vi "Bertta_v09_91.vi"() -> ()   [LabVIEW 2015]
panel:
  out "element":bool
  out "Started:":string
  in  "SHUTDOWN":bool
  in  "MASTER CONTROL":bool
  in  "Tab Control":T1(tab)
  out "Output File":path caption="selected path"
  in  "Browse folder":path=path "" caption="start path"
  in  "Read Seq":bool
  in  "Save Seq":bool
  in  "Configuration file":path=path "C:/Users/shresplab/Desktop/BerttaConfiguration.lvm" caption="Filename"
  in  "OK Button 2":bool
  out "Boolean":bool
  in  "User (initials)":string
  in  "Project name":string
  in  "Description":string
  out "PUMP1":bool
  out "Target amount":dbl
  out "Scale weight":dbl
  out "Amount now":dbl
  out "Flow rate":dbl
  out "Time to target":dbl format="%<%H:%M:%S>t"
  out "Current step":dbl
  out "Target":dbl
  out "Amount now":dbl
  out "Amount now":dbl
  out "Target":dbl
  out "Current step":dbl
  out "Time to target":dbl format="%<%H:%M:%S>t"
  out "Flow rate":dbl
  out "Amount now":dbl
  out "Scale weight":dbl
  out "Target amount":dbl
  out "PUMP2":bool
  out "Sensor OK 6":bool
  out "Sensor OK 5":bool
  out "Sensor OK 4":bool
  out "Sensor OK 3":bool
  in  "OK Button":bool
  in  "Add comment":string
  out "PUMP3":bool
  out "Target amount":dbl
  out "Scale weight":dbl
  out "Amount now":dbl
  out "Flow rate":dbl
  out "Time to target":dbl format="%<%H:%M:%S>t"
  out "Current step":dbl
  out "Target":dbl
  out "Amount now":dbl
  out "Tr":dbl
  out "Tj in":dbl
  out "Tj out":dbl
  out "T set":dbl
  out "Current step":i32
  out "RPM":dbl
  out "Torque 2":dbl
  out "Waveform Chart 5":dynamicdata(graph)
  out "Waveform Chart 6":dynamicdata(graph)
  out "Waveform Chart 7":dynamicdata(graph)
  in  "Tab Control 2":T2(tab)
  out "Waveform Chart 3":dynamicdata(graph)
  out "Waveform Chart 8":dynamicdata(graph)
  out "Waveform Chart 11":dynamicdata(graph)
  out "Waveform Chart 13":dynamicdata(graph)
  out "Waveform Chart 9":dynamicdata(graph)
  out "Table":string[][](table)=[["14.8.2017 18.06.59", "0,000000", "417,670000", "-0,150000", "1,000000", "22,220000", "23,366837", "23,574959", "23,985852", "23,690000", "240,000000", "4,000000", "0,000000", "397,000000", "-397,000000", "1,000000"], ["14.8.2017 18.07.06", "0,000000", "417,640000", "-0,120000", "1,000000", "22,220000", "23,763115", "23,906257", "23,985694", "23,680000", "240,000000", "4,000000", "0,000000", "397,000000", "-397,000000", "1,000000"], ["14.8.2017 18.07.13", "0,000000", "417,640000", "-0,120000", "1,000000", "22,220000", "23,965922", "24,013440", "23,984906", "23,670000", "240,000000", "4,100000", "3,000000", "397,000000", "-397,000000", "1,000000"], ["14.8.2017 18.07.21", "0,000000", "417,640000", "-0,120000", "1,000000", "22,220000", "23,943860", "23,900110", "23,987113", "23,670000", "240,000000", "4,000000", "0,000000", "397,000000", "-397,000000", "1,000000"], ["14.8.2017 18.07.28", "0,000000", "417,640000", "-0,120000", "1,000000", "22,220000", "23,736328", "23,600018", "23,989004", "23,660000", "240,000000", "4,000000", "0,000000", "397,000000", "-397,000000", "1,000000"], ["14.8.2017 18.07.36", "0,000000", "417,640000", "-0,120000", "1,000000", "22,220000", "23,480910", "23,324538", "23,991053", "23,660000", "240,000000", "4,000000", "0,000000", "397,000000", "-397,000000", "1,000000"], ["14.8.2017 18.07.43", "0,000000", "417,640000", "-0,120000", "2,000000", "22,220000", "23,195579", "23,008270", "23,999093", "23,650000", "240,000000", "4,000000", "0,000000", "397,000000", "-397,000000", "1,000000"], ["14.8.2017 18.07.51", "0,000000", "417,650000", "-417,650000", "1,000000", "22,220000", "22,862541", "22,649021", "24,003979", "23,650000", "240,000000", "4,000000", "0,000000", "397,000000", "-397,000000", "2,000000"], ["14.8.2017 18.07.58", "0,000000", "417,640000", "0,010000", "1,000000", "22,220000", "22,541353", "22,354878", "24,005398", "23,650000", "240,000000", "4,000000", "0,000000", "397,000000", "-397,000000", "1,000000"], ["14.8.2017 18.08.06", "0,000000", "417,640000", "0,010000", "1,000000", "22,220000", "22,347931", "22,253738", "24,007605", "23,640000", "240,000000", "4,100000", "0,000000", "397,000000", "-397,000000", "1,000000"], ["14.8.2017 18.08.13", "0,000000", "417,640000", "0,010000", "1,000000", "22,220000", "22,329030", "22,302102", "24,006028", "23,640000", "240,000000", "4,000000", "0,000000", "395,820000", "-395,820000", "1,000000"], ["14.8.2017 18.08.20", "0,000000", "417,640000", "0,010000", "1,000000", "22,220000", "22,466849", "22,511320", "24,002403", "23,630000", "240,000000", "4,000000", "0,000000", "395,830000", "-0,010000", "1,000000"], ["14.8.2017 18.08.28", "0,000000", "417,640000", "0,010000", "1,000000", "22,220000", "22,707062", "22,835101", "24,000984", "23,620000", "240,000000", "4,000000", "0,000000", "395,830000", "-0,010000", "1,000000"], ["14.8.2017 18.08.35", "0,000000", "417,640000", "0,010000", "1,000000", "22,220000", "23,054104", "23,232979", "24,001299", "23,600000", "240,000000", "4,000000", "0,000000", "395,830000", "-0,010000", "1,000000"], ["14.8.2017 18.08.43", "0,000000", "417,640000", "0,010000", "1,000000", "22,220000", "23,412371", "23,522793", "24,002560", "23,590000", "240,000000", "4,000000", "0,000000", "395,820000", "0,000000", "1,000000"], ["14.8.2017 18.08.51", "0,000000", "417,640000", "0,010000", "1,000000", "22,220000", "23,596247", "23,656125", "24,003821", "23,580000", "240,000000", "4,000000", "0,000000", "395,820000", "0,000000", "1,000000"]]
  out "Boolean 2":bool
  in  "Time":dbl format="Time to target (min):                %#_g"
  out "Current temp":dbl format="Current temperature (S1):   %#_6g"
  in  "OK Button 3":bool
  in  "T ext / T ext 2":enum32{"Sensor 1", "Sensor 2"}(radio)
  out "Sensor OK":bool
  in  "T fail":dbl=20.0 format="Failsafe temperature:              %#_g"
  in  "Setpoint":dbl=20.0 format="Temperature target:                %#_6g"
  in  "Manual select":T3(radio)
  in  "PAUSE":bool
  out "Waveform Chart":dynamicdata(graph)
  out "T external 2":dbl format="Current temperature (S2):    %#_g"
  out "Led11 5":bool
  out "RPM":dbl format="%_4f"
  out "Led10 3":bool
  out "Led9 3":bool
  out "Led8 3":bool
  out "Led7 3":bool
  out "Led6 3":bool
  out "Led5 3":bool
  out "Led4 3":bool
  out "Led3 3":bool
  out "Led2 3":bool
  out "Led1 3":bool
  in  "PumpSeq 4":dbl[][](array[numeric])=[[1.0, 1.0, 0.0, 0.0, 0.0, 0.0, 0.0, 0.0, 0.0, 0.0], [2.0, 1.0, 0.0, 0.0, 0.0, 0.0, 0.0, 0.0, 0.0, 0.0], [3.0, 1.0, 0.0, 0.0, 0.0, 0.0, 0.0, 0.0, 0.0, 0.0], [0.0, 0.0, 0.0, 0.0, 0.0, 0.0, 0.0, 0.0, 0.0, 0.0], [0.0, 0.0, 0.0, 0.0, 0.0, 0.0, 0.0, 0.0, 0.0, 0.0], [0.0, 0.0, 0.0, 0.0, 0.0, 0.0, 0.0, 0.0, 0.0, 0.0], [0.0, 0.0, 0.0, 0.0, 0.0, 0.0, 0.0, 0.0, 0.0, 0.0], [0.0, 0.0, 0.0, 0.0, 0.0, 0.0, 0.0, 0.0, 0.0, 0.0], [0.0, 0.0, 0.0, 0.0, 0.0, 0.0, 0.0, 0.0, 0.0, 0.0], [0.0, 0.0, 0.0, 0.0, 0.0, 0.0, 0.0, 0.0, 0.0, 0.0]]
  in  "?":bool
  out "Flow rate (g/min)":dbl
  out "Scale reading":dbl
  out "Step amount now":dbl
  in  "Grams / min":dbl
  out "Waveform Chart 14":dynamicdata(graph)
  in  "?":bool
  out "Total amount now":dbl
  out "Led11 4":bool
  in  "Reset 5":bool
  out "Elapsed / step":i32
  out "Time to target":dbl format="%<%H:%M:%S>t"
  in  "OK Button 4":bool
  out "Led11":bool
  out "RPM":dbl format="%_4f"
  out "Led10":bool
  out "Led9":bool
  out "Led8":bool
  out "Led7":bool
  out "Led6":bool
  out "Led5":bool
  out "Led4":bool
  out "Led3":bool
  out "Led2":bool
  out "Led1":bool
  in  "PumpSeq 2":dbl[][](array[numeric])=[[1.0, 2.0, 0.0, 0.0, 0.0, 0.0, 0.0, 0.0, 0.0, 0.0], [2.0, 2.0, 0.0, 0.0, 0.0, 0.0, 0.0, 0.0, 0.0, 0.0], [3.0, 2.0, 0.0, 0.0, 0.0, 0.0, 0.0, 0.0, 0.0, 0.0], [0.0, 0.0, 0.0, 0.0, 0.0, 0.0, 0.0, 0.0, 0.0, 0.0], [0.0, 0.0, 0.0, 0.0, 0.0, 0.0, 0.0, 0.0, 0.0, 0.0], [0.0, 0.0, 0.0, 0.0, 0.0, 0.0, 0.0, 0.0, 0.0, 0.0], [0.0, 0.0, 0.0, 0.0, 0.0, 0.0, 0.0, 0.0, 0.0, 0.0], [0.0, 0.0, 0.0, 0.0, 0.0, 0.0, 0.0, 0.0, 0.0, 0.0], [0.0, 0.0, 0.0, 0.0, 0.0, 0.0, 0.0, 0.0, 0.0, 0.0], [0.0, 0.0, 0.0, 0.0, 0.0, 0.0, 0.0, 0.0, 0.0, 0.0]]
  in  "?":bool
  out "Flow rate (g/min)":dbl
  out "Scale reading":dbl
  out "Step amount now":dbl
  in  "Grams / min":dbl
  out "Waveform Chart 10":dynamicdata(graph)
  in  "?":bool
  out "Total amount now":dbl
  out "Led11":bool
  in  "Reset 3":bool
  out "Elapsed / step":i32
  out "Time to target":dbl format="%<%H:%M:%S>t"
  in  "OK Button 5":bool
  out "Led11 3":bool
  out "RPM":dbl format="%_4f"
  out "Led10 2":bool
  out "Led9 2":bool
  out "Led8 2":bool
  out "Led7 2":bool
  out "Led6 2":bool
  out "Led5 2":bool
  out "Led4 2":bool
  out "Led3 2":bool
  out "Led2 2":bool
  out "Led1 2":bool
  in  "PumpSeq 3":dbl[][](array[numeric])=[[1.0, 3.0, 0.0, 0.0, 0.0, 0.0, 0.0, 0.0, 0.0, 0.0], [2.0, 3.0, 0.0, 0.0, 0.0, 0.0, 0.0, 0.0, 0.0, 0.0], [3.0, 3.0, 0.0, 0.0, 0.0, 0.0, 0.0, 0.0, 0.0, 0.0], [0.0, 0.0, 0.0, 0.0, 0.0, 0.0, 0.0, 0.0, 0.0, 0.0], [0.0, 0.0, 0.0, 0.0, 0.0, 0.0, 0.0, 0.0, 0.0, 0.0], [0.0, 0.0, 0.0, 0.0, 0.0, 0.0, 0.0, 0.0, 0.0, 0.0], [0.0, 0.0, 0.0, 0.0, 0.0, 0.0, 0.0, 0.0, 0.0, 0.0], [0.0, 0.0, 0.0, 0.0, 0.0, 0.0, 0.0, 0.0, 0.0, 0.0], [0.0, 0.0, 0.0, 0.0, 0.0, 0.0, 0.0, 0.0, 0.0, 0.0], [0.0, 0.0, 0.0, 0.0, 0.0, 0.0, 0.0, 0.0, 0.0, 0.0]]
  in  "?":bool
  out "Flow rate (g/min)":dbl
  out "Scale reading":dbl
  out "Step amount now":dbl
  in  "Grams / min":dbl
  out "Waveform Chart 12":dynamicdata(graph)
  in  "?":bool
  out "Total amount now":dbl
  out "Led11 2":bool
  in  "Reset 4":bool
  out "Elapsed / step":i32
  out "Time to target":dbl format="%<%H:%M:%S>t"
  in  "OK Button 6":bool
  in  "Bypass select 2":enum32{"Remote", "Manual"}(radio)=enum."Manual"
  in  "Port":dbl=13.0
  out "RPM":dbl
  out "Torque":dbl
  in  "Set RPM":dbl(slide) scale=0.0..2000.0
  out "Waveform Chart 4":dynamicdata(graph)
  in  "OK Button 7":bool
  in  "Treshold (T/C)":dbl=0.5
  out "DAQ 9217 (PT100)":errorcluster
  out "Config File":dbl[][](array[numeric])
  # "Temperature sensor:"
  # "Manual control:"
  # "PUMP & SCALE 1"
  # "STEP"
  # "TOTAL"
  # "PUMP & SCALE 2"
  # "STEP"
  # "TOTAL"
  # "PUMP & SCALE 3"
  # "STEP"
  # "TOTAL"
  # "Temperature control parameter"
  # "Secondary temperature sensor"
  # "Grams    /   min"
  # "End of sequence"
  # "Manual control"
  # "Grams    /   min"
  # "End of sequence"
  # "Manual control"
  # "Grams    /   min"
  # "End of sequence"
  # "Manual control"
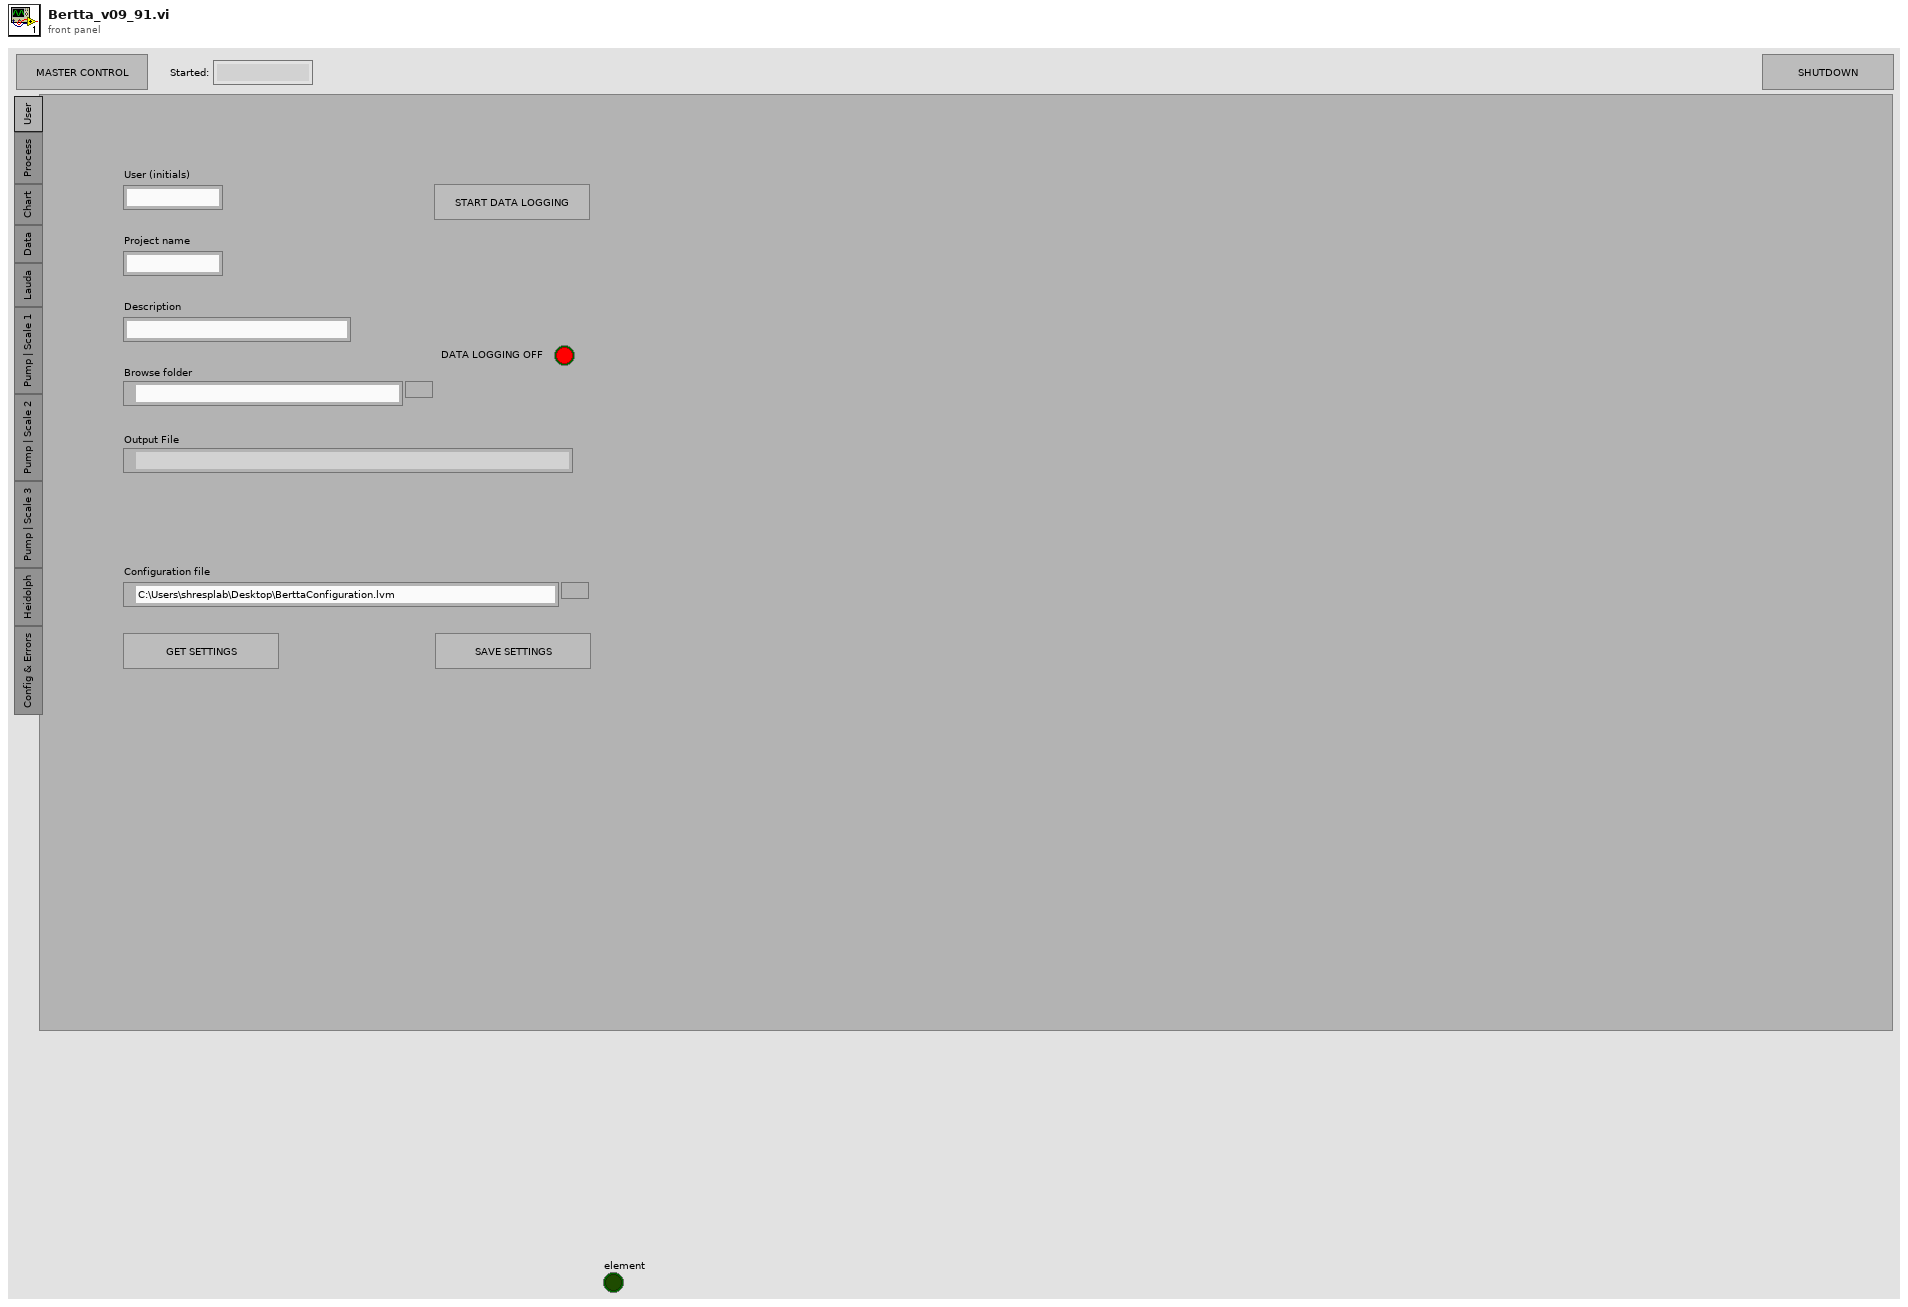
[diagram p1: front panel]
types:
  T1 = enum32{"User", "Process", "Chart", "Data", "Lauda", "Pump | Scale 1", "Pump | Scale 2", "Pump | Scale 3", "Heidolph", "Config & Errors"}
  T2 = enum32{"Temperatures", "Scale / Pump 1", "Scale / Pump 2", "Scale / Pump 3", "RPM / torque"}
  T3 = enum32{"Reactor temperature", "Jacket temperature"}
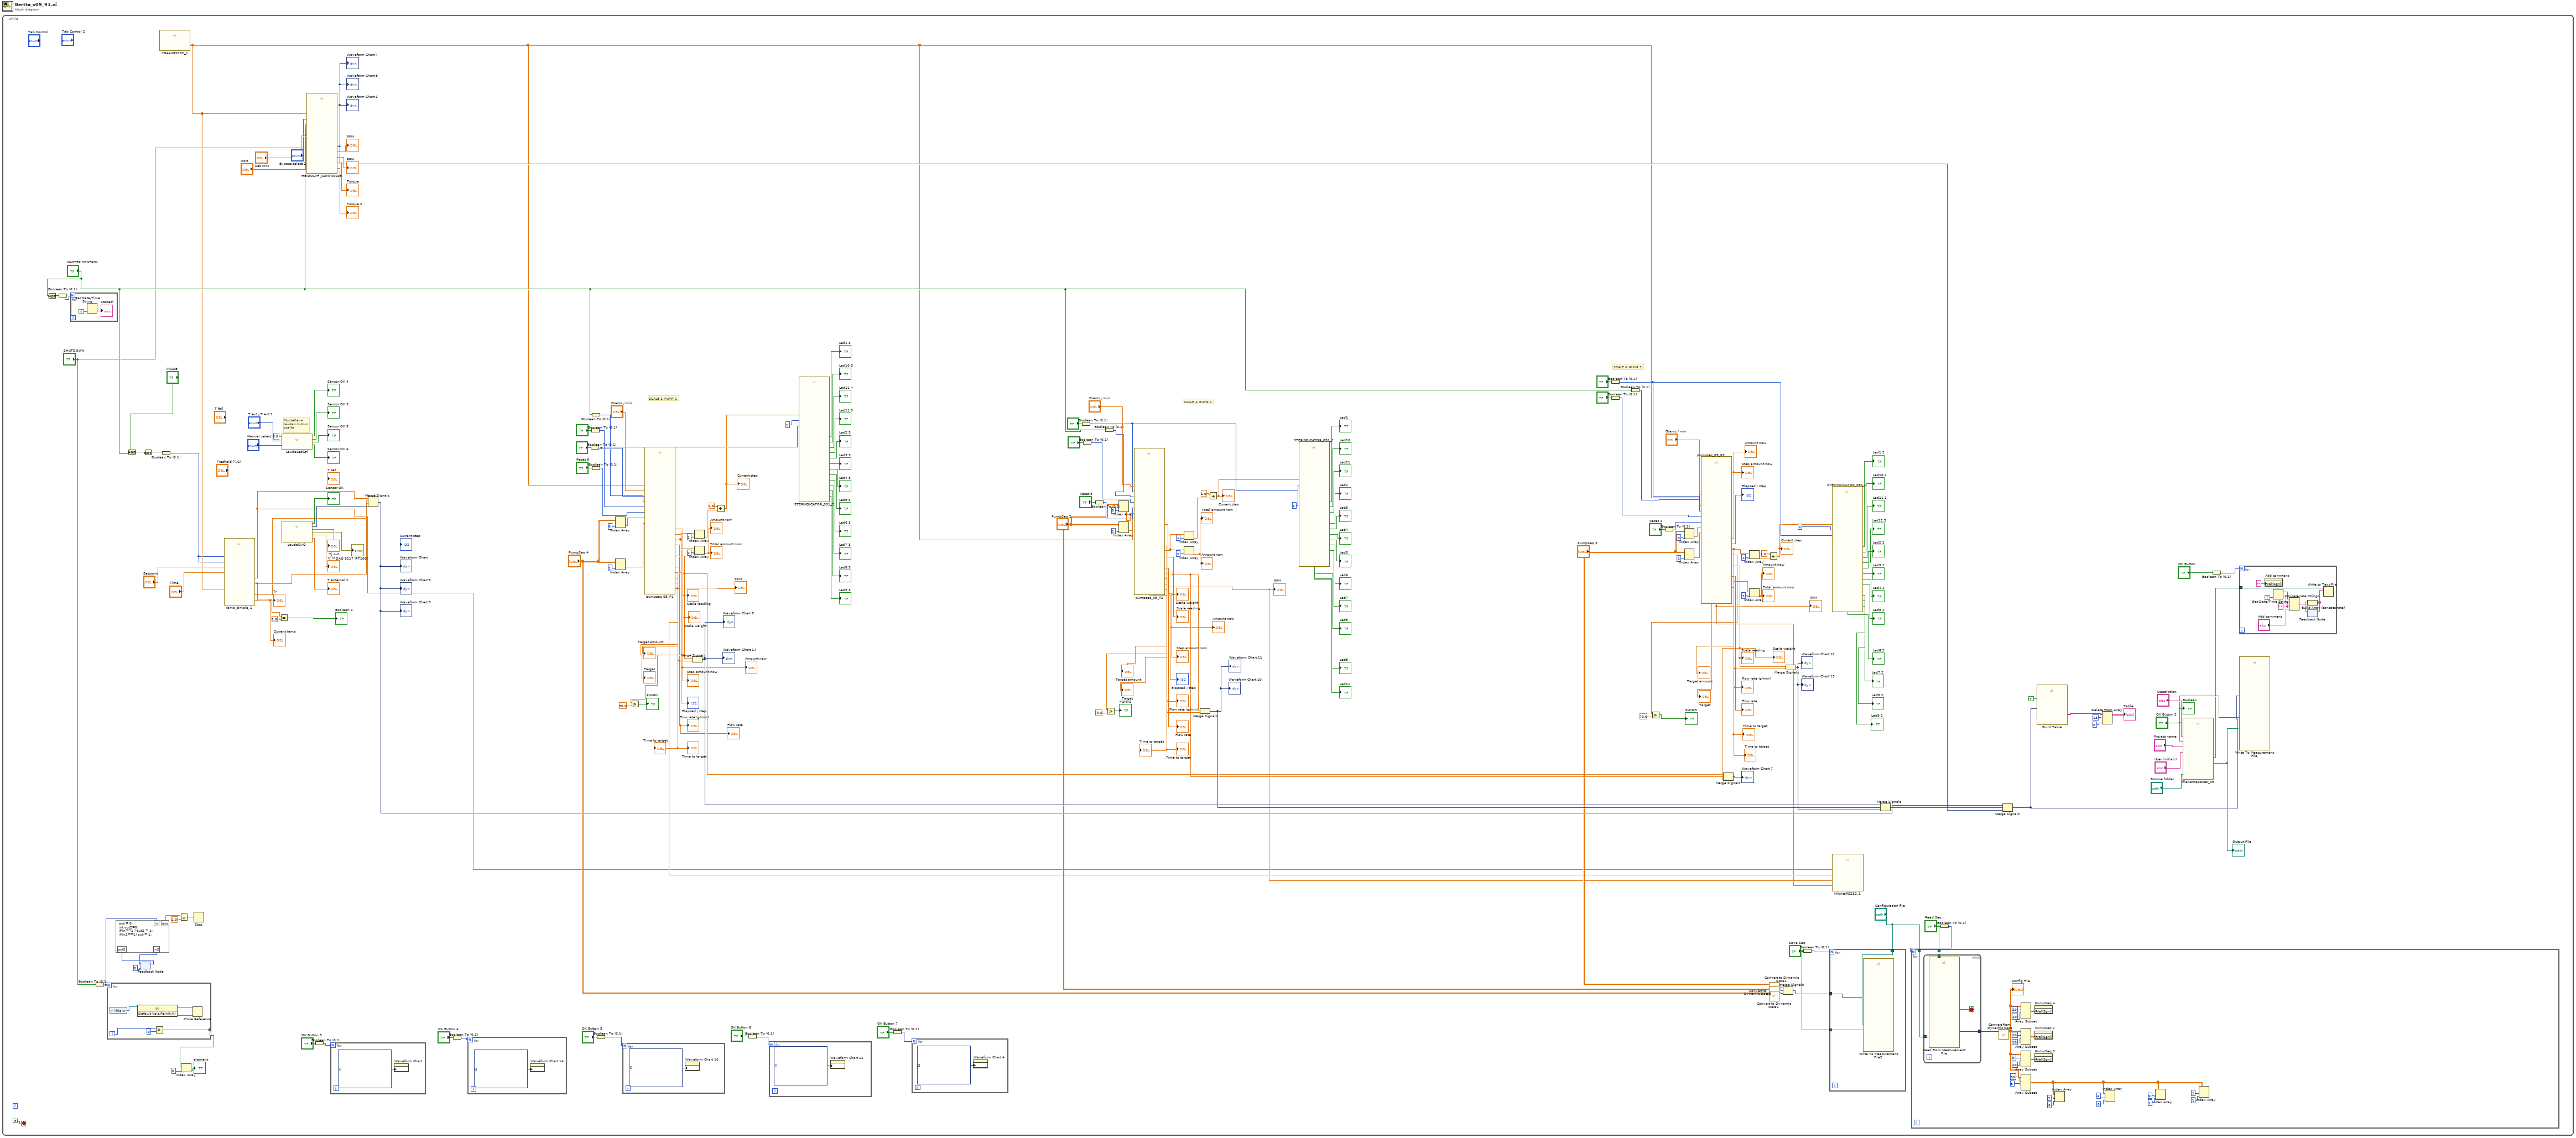
[diagram p0: block diagram]
diagram:
  n1 = while {
    stop <- FALSE stop-if-true
    # "Muutettava\nlaudan kutsun \nosalta"
    # "SCALE & PUMP 1"
    # "SCALE & PUMP 3"
    # "SCALE & PUMP 2"
    n2 = Not(x="MASTER CONTROL") -> (.not. x?=w210:bool)
    n3 = Boolean To (0,1)(Boolean=w210) -> (0, 1=w211:i16)
    n4 = for {
      N: w211 -> [_]
      n5 = Get Date/Time String(want seconds? (F)=TRUE) -> (time string=→"Started:":string)  [unwired: 2 in, 1 out]
    }
    n6 = Boolean To (0,1)(Boolean="SHUTDOWN") -> (0, 1=w193:i16)
    n7 = for {
      N: w193 -> [_]
      tunnel: [w268] -> w209 mode=indexing
      i -> [w270]
      n8 = control-ref of="This VI"() -> (w273:refnum<vi>)
      n9 = invoke class="VI" method="Default Vals.Reinit All"(reference=w273) -> (reference out=w271:refnum<vi>, error out=w272:errorcluster)  [unwired: 2 in, 1 out]
      n10 = Greater?(x=w270, y=0) -> (0:w268:bool)
      n11 = Close Reference(reference=w271, error in (no error)=w272) -> ()  [unwired: 1 out]
    }
    n12 = And(x="PAUSE", y="MASTER CONTROL") -> (x .and. y?=w156:bool)
    n13 = feedback #1(0) -> (w191:i32)
    n14 = formula code="out = 0;\nint out2=0;\nif(in==1 ) out2 = 1;\nif(in2==1) out = 1;"("in"=w193, "in2"=w191) -> ("out"=w195:dbl, "out2"=w192:i32)
    n15 = feedback-in #1(w192) -> ()
    n16 = Not(x=w156) -> (.not. x?=w11:bool)
    n17 = call "MReadRS232_1.vi"() -> ("params"=w8:dbl[])  [unwired: 11 in]
    n18 = Boolean To (0,1)(Boolean=w11) -> (0, 1=w4:i16)
    n19 = Equal?(x=w195, y=1.0) -> (x = y?=w194:bool)
    n20 = Index Array(array=w209, index=0) -> (element=→"element":bool)
    n21 = Stop(stop? (T)=w194) -> ()
    n22 = call "ramp_simple_1.vi"("array"=w8, "time_set"="Time", "T_sp"="Setpoint", "reset"=w4, "pause"=w4) -> ("T control"=w7:dbl, "Tr"=w6:dbl, "Tin"=w5:dbl, "reset_out"=w2:dbl)  [unwired: 3 in]
    "Tr" <- w6
    "Current temp" <- w6
    n23 = Equal?(x=w2, y=1.0) -> (x = y?=→"Boolean 2":bool)
    n24 = call "LaudaLedCtrl.vi"("Manual select"="Manual select", "T ext / T ext in"="T ext / T ext 2", "Lauda port"=9.0) -> ("Sensor OK 5"=→"Sensor OK 5":bool, "Sensor OK 3"=→"Sensor OK 3":bool, "Sensor OK 4"=→"Sensor OK 4":bool, "Sensor OK 6"=→"Sensor OK 6":bool)  [unwired: 5 in]
    n25 = call "LaudaDAQ.vi"() -> ("error out"=→"DAQ 9217 (PT100)":errorcluster, 1:"Tj out"=→"Tj out":dbl, "data"=w79:dynamicdata, "Sensor OK"=→"Sensor OK":bool, 4:"Tj out"=→"Tj in":dbl, "T external 2"=→"T external 2":dbl)  [unwired: 6 in]
    n26 = call "HEIDOLPH_CONTROL09.vi"("master"="MASTER CONTROL", "Array"=w8, "shutdown"="SHUTDOWN", "Bypass select"="Bypass select 2", "Set RPM"="Set RPM", "Device port"="Port") -> ("Dynamic Data"=w80:dynamicdata, "RPM"=→"RPM":dbl, "RPM 2"=→"RPM":dbl, "Torque"=→"Torque":dbl, "Torque 2"=→"Torque 2":dbl)  [unwired: 1 in]
    "Waveform Chart 4" <- w80
    "Waveform Chart 6" <- w80
    "Waveform Chart 9" <- w80
    n27 = Boolean To (0,1)(Boolean="OK Button 3") -> (0, 1=w22:i16)
    n28 = for {
      N: w22 -> [_]
      n29 = property on="Waveform Chart" class="WFChart (strict)"("History Data"=dynamicdata[] []) -> ()  [unwired: 2 in, 2 out]
    }
    n30 = Merge Signals(w7, w6, w5, w79) -> (w81:dynamicdata)
    "Waveform Chart 3" <- w81
    "Waveform Chart" <- w81
    "Waveform Chart 5" <- w81
    n31 = Boolean To (0,1)(Boolean="OK Button 4") -> (0, 1=w20:i16)
    n32 = for {
      N: w20 -> [_]
      n33 = property on="Waveform Chart 14" class="WFChart (strict)"("History Data"=dynamicdata[] []) -> ()  [unwired: 2 in, 2 out]
    }
    n34 = Boolean To (0,1)(Boolean="?") -> (0, 1=w90:i16)
    n35 = Boolean To (0,1)(Boolean="?") -> (0, 1=w94:i16)
    n36 = Boolean To (0,1)(Boolean="MASTER CONTROL") -> (0, 1=w86:i16)
    n37 = Boolean To (0,1)(Boolean="Reset 5") -> (0, 1=w93:i16)
    n38 = Boolean To (0,1)(Boolean="OK Button 5") -> (0, 1=w18:i16)
    n39 = Index Array(array="PumpSeq 4", index (col)=0) -> (element=w98:dbl[])  [unwired: 1 in]
    n40 = Index Array(array="PumpSeq 4", index (col)=1) -> (element=w119:dbl[])  [unwired: 1 in]
    n41 = for {
      N: w18 -> [_]
      n42 = property on="Waveform Chart 10" class="WFChart (strict)"("History Data"=dynamicdata[] []) -> ()  [unwired: 2 in, 2 out]
    }
    n43 = call "pumpsec_09_P1.vi"("reset"=w93, "master"=w86, "manual"=w90, "pause"=w94, "Array"=w8, "Target"=w98, "fr_manual"="Grams / min", "Time"=w119) -> ("pumpCtrl"=w63:dbl, "totaltarget"=→"Target":dbl, "target_step"=→"Target amount":dbl, "REGLO D"=w29:dbl, "time_to_target"=→"Time to target" →"Time to target":dbl, "step_fr"=w40:dbl, "amount_step"=→"Amount now" →"Step amount now":dbl, "Scale"=w75:dbl, "elapsed_step"=→"Elapsed / step":dbl, "params"=w116:dbl[])  [unwired: 8 in, 2 out]
    "Flow rate" <- w40
    "Scale weight" <- w75
    "Scale reading" <- w75
    "Flow rate (g/min)" <- w40
    "RPM" <- w29
    n44 = Greater?(x=w63, y=70.0) -> (0:→"PUMP1":bool)
    n45 = Merge Signals(w75, w40) -> (w84:dynamicdata)
    "Waveform Chart 8" <- w84
    "Waveform Chart 14" <- w84
    n46 = Index Array(array=w116, index=1) -> (element=w113:dbl)
    n47 = Index Array(array=w116, index=2) -> (element=→"Amount now" →"Total amount now":dbl)
    n48 = Add(x=1.0, y=w113) -> (x+y=w41:dbl)
    "Current step" <- w41
    n49 = Boolean To (0,1)(Boolean="OK Button 6") -> (0, 1=w16:i16)
    n50 = for {
      N: w16 -> [_]
      n51 = property on="Waveform Chart 12" class="WFChart (strict)"("History Data"=dynamicdata[] []) -> ()  [unwired: 2 in, 2 out]
    }
    n52 = call "STEPINDICATOR_091_2.vi"("current step"=w41, "enable"=i16 1, "manual"=w90) -> ("Led 8"=→"Led8 3":bool, "Led 10"=→"Led10 3":bool, "Led 11"=→"Led11 4":bool, "Led 7"=→"Led7 3":bool, "Led 1"=→"Led1 3":bool, "Led 6"=→"Led6 3":bool, "Led 2"=→"Led2 3":bool, "Led 12"=→"Led11 5":bool, "Led 5"=→"Led5 3":bool, "Led 4"=→"Led4 3":bool, "Led 3"=→"Led3 3":bool, "Led 9"=→"Led9 3":bool)  [unwired: 1 in]
    n53 = Boolean To (0,1)(Boolean="OK Button 7") -> (0, 1=w14:i16)
    n54 = for {
      N: w14 -> [_]
      n55 = property on="Waveform Chart 4" class="WFChart (strict)"("History Data"=dynamicdata[] []) -> ()  [unwired: 2 in, 2 out]
    }
    n56 = Boolean To (0,1)(Boolean="?") -> (0, 1=w153:i16)
    n57 = Boolean To (0,1)(Boolean="?") -> (0, 1=w182:i16)
    n58 = Boolean To (0,1)(Boolean="Reset 3") -> (0, 1=w180:i16)
    n59 = Boolean To (0,1)(Boolean="MASTER CONTROL") -> (0, 1=w174:i16)
    n60 = Index Array(array="PumpSeq 2", index (col)=0 ("disabled index (col)")) -> (element=w185:dbl[])  [unwired: 1 in]
    n61 = Index Array(array="PumpSeq 2", index (col)=1 ("disabled index (col)")) -> (element=w184:dbl[])  [unwired: 1 in]
    n62 = call "pumpsec_09_P2.vi"("reset"=w180, "master"=w174, "manual"=w153, "pause"=w182, "Array"=w8, "Target"=w185, "fr_manual"="Grams / min", "Time"=w184) -> ("pumpCtrl"=w59:dbl, "totaltarget"=→"Target":dbl, "target_step"=→"Target amount":dbl, "REGLO D"=w28:dbl, "time_to_target"=→"Time to target" →"Time to target":dbl, "step_fr"=w78:dbl, "amount_step"=→"Amount now" →"Step amount now":dbl, "Scale"=w74:dbl, "elapsed_step"=→"Elapsed / step":dbl, "params"=w175:dbl[])  [unwired: 8 in, 2 out]
    "Scale weight" <- w74
    "Flow rate" <- w78
    "Scale reading" <- w74
    "Flow rate (g/min)" <- w78
    "RPM" <- w28
    n63 = Greater?(x=w59, y=70.0) -> (0:→"PUMP2":bool)
    n64 = Index Array(array=w175, index=1) -> (element=w178:dbl)
    n65 = Index Array(array=w175, index=2) -> (element=→"Amount now" →"Total amount now":dbl)
    n66 = Merge Signals(w74, w78) -> (w87:dynamicdata)
    "Waveform Chart 11" <- w87
    "Waveform Chart 10" <- w87
    n67 = Add(x=1.0, y=w178) -> (x+y=w172:dbl)
    "Current step" <- w172
    n68 = call "STEPINDICATOR_091_2.vi"("current step"=w172, "enable"=i16 1, "manual"=w153) -> ("Led 8"=→"Led8":bool, "Led 10"=→"Led10":bool, "Led 11"=→"Led11":bool, "Led 7"=→"Led7":bool, "Led 1"=→"Led1":bool, "Led 6"=→"Led6":bool, "Led 2"=→"Led2":bool, "Led 12"=→"Led11":bool, "Led 5"=→"Led5":bool, "Led 4"=→"Led4":bool, "Led 3"=→"Led3":bool, "Led 9"=→"Led9":bool)  [unwired: 1 in]
    n69 = Boolean To (0,1)(Boolean="?") -> (0, 1=w147:i16)
    n70 = Boolean To (0,1)(Boolean="?") -> (0, 1=w146:i16)
    n71 = Boolean To (0,1)(Boolean="MASTER CONTROL") -> (0, 1=w148:i16)
    n72 = Boolean To (0,1)(Boolean="Reset 4") -> (0, 1=w128:i16)
    n73 = Index Array(array="PumpSeq 3", index (col)=0 ("disabled index (col)")) -> (element=w131:dbl[])  [unwired: 1 in]
    n74 = Index Array(array="PumpSeq 3", index (col)=1 ("disabled index (col)")) -> (element=w130:dbl[])  [unwired: 1 in]
    n75 = call "pumpsec_09_P3.vi"("reset"=w128, "master"=w148, "manual"=w147, "pause"=w146, "Array"=w8, "Target"=w131, "fr_manual"="Grams / min", "Time"=w130) -> ("pumpCtrl"=w56:dbl, "totaltarget"=→"Target":dbl, "target_step"=→"Target amount":dbl, "REGLO D"=w27:dbl, "time_to_target"=→"Time to target" →"Time to target":dbl, "step_fr"=w77:dbl, "amount_step"=→"Amount now" →"Step amount now":dbl, "Scale"=w73:dbl, "elapsed_step"=→"Elapsed / step":dbl, "params"=w121:dbl[])  [unwired: 8 in, 2 out]
    "Scale weight" <- w73
    "Flow rate" <- w77
    "Scale reading" <- w73
    "Flow rate (g/min)" <- w77
    "RPM" <- w27
    n76 = Greater?(x=w56, y=70.0) -> (0:→"PUMP3":bool)
    n77 = Merge Signals(w75, w74, w73) -> (→"Waveform Chart 7":dynamicdata)
    n78 = Index Array(array=w121, index=1) -> (element=w122:dbl)
    n79 = Index Array(array=w121, index=2) -> (element=→"Amount now" →"Total amount now":dbl)
    n80 = Add(x=1.0, y=w122) -> (x+y=w120:dbl)
    "Current step" <- w120
    n81 = call "Convert to Dynamic Data4"("2D Array"="PumpSeq 3") -> ("Dynamic Data Type"=w32:dynamicdata)  [unwired: 3 in]
    n82 = call "Convert to Dynamic Data3"("2D Array"="PumpSeq 2") -> ("Dynamic Data Type"=w34:dynamicdata)  [unwired: 3 in]
    n83 = call "Convert to Dynamic Data2"("2D Array"="PumpSeq 4") -> ("Dynamic Data Type"=w37:dynamicdata)  [unwired: 3 in]
    n84 = Merge Signals(w32, w34, w37) -> (w36:dynamicdata)
    n85 = Merge Signals(w73, w77) -> (w83:dynamicdata)
    "Waveform Chart 13" <- w83
    "Waveform Chart 12" <- w83
    n86 = Boolean To (0,1)(Boolean="Save Seq") -> (0, 1=w31:i16)
    n87 = for {
      N: w31 -> [_]
      tunnel: w36 -> [w266]
      tunnel: "Configuration file" -> [w267]
      tunnel: "Save Seq" -> [w265]
      n88 = call "Write To Measurement File2"("Signals"=w266, "Reset"=w265, "Filename"=w267) -> ()  [unwired: 14 in, 3 out]
    }
    n89 = call "STEPINDICATOR_091_4.vi"("current step"=w120, "enable"=i16 1, "manual"=w147) -> ("Led 8"=→"Led8 2":bool, "Led 10"=→"Led10 2":bool, "Led 11"=→"Led11 2":bool, "Led 7"=→"Led7 2":bool, "Led 1"=→"Led1 2":bool, "Led 6"=→"Led6 2":bool, "Led 2"=→"Led2 2":bool, "Led 12"=→"Led11 3":bool, "Led 5"=→"Led5 2":bool, "Led 4"=→"Led4 2":bool, "Led 3"=→"Led3 2":bool, "Led 9"=→"Led9 2":bool)  [unwired: 1 in]
    n90 = call "MWriteRS232_1.vi"("P3"=w27, "P2"=w28, "P1"=w29, "LAUDA"=w7) -> ()  [unwired: 8 in]
    n91 = Merge Signals(w84, w87, w83) -> (w82:dynamicdata)
    n92 = Boolean To (0,1)(Boolean="Read Seq") -> (0, 1=w30:i16)
    n93 = for {
      N: w30 -> [_]
      tunnel: "Configuration file" -> [w238]
      tunnel: "Read Seq" -> [w237]
      n94 = while {
        tunnel: [w264] -> w260
        tunnel: w238 -> [w263]
        tunnel: w237 -> [w261]
        stop <- w262 stop-if-true
        n95 = call "Read From Measurement File"("Filename"=w263, "Reset"=w261) -> ("Signals"=w264:dynamicdata, "EOF?"=w262:bool)  [unwired: 4 in, 4 out]
      }
      n96 = call "Convert from Dynamic Data"("Dynamic Data Type"=w260) -> ("Array"=w250:dbl[][])  [unwired: 3 in]
      "Config File" <- w250
      n97 = Array Subset(array=w250, index (row)=20 ("index"), length (row)=10 ("length")) -> (w257:dbl[][])  [unwired: 2 in]
      n98 = Array Subset(array=w250, index (row)=10 ("index"), length (row)=10 ("length")) -> (w252:dbl[][])  [unwired: 2 in]
      n99 = Array Subset(array=w250, index (row)=0 ("index"), length (row)=10 ("length")) -> (w251:dbl[][])  [unwired: 2 in]
      n100 = Array Subset(array=w250, index (row)=30 ("index"), length (row)=8 ("length")) -> (w239:dbl[][])  [unwired: 2 in]
      n101 = property on="PumpSeq 4" class="Arr (strict)"("Val(Sgnl)"=w257) -> ()  [unwired: 2 in, 2 out]
      n102 = property on="PumpSeq 2" class="Arr (strict)"("Val(Sgnl)"=w252) -> ()  [unwired: 2 in, 2 out]
      n103 = property on="PumpSeq 3" class="Arr (strict)"("Val(Sgnl)"=w251) -> ()  [unwired: 2 in, 2 out]
      n104 = Index Array(array=w239, index (row)=2, index (col)=0 ("disabled index (col)")) -> ()  [unwired: 1 out]
      n105 = Index Array(array=w239, index (row)=4, index (col)=0 ("disabled index (col)")) -> ()  [unwired: 1 out]
      n106 = Index Array(array=w239, index (row)=0, index (col)=1 ("disabled index (col)")) -> ()  [unwired: 1 out]
      n107 = Index Array(array=w239, index (row)=1, index (col)=1 ("disabled index (col)")) -> ()  [unwired: 1 out]
    }
    n108 = Merge Signals(w81, w82, w80) -> (w204:dynamicdata)
    n109 = call "Build Table"("Include time data"=TRUE, "Signals"=w204) -> ("Table"=w203:string[][])  [unwired: 3 in, 6 out]
    n110 = Delete From Array(array=w203, length=13, index (col)=0 ("index (row)")) -> (array with subset deleted=→"Table":string[][])  [unwired: 1 in, 1 out]
    n111 = call "filenameparser_09.vi"("Description"="Description", "start path"="Browse folder", "Project name"="Project name", "User (initials)"="User (initials)", "OK Button in"="OK Button 2") -> ("appended path 2"=w12:path, "appended path"=w199:path)  [unwired: 4 in, 1 out]
    "Output File" <- w12
    n112 = Boolean To (0,1)(Boolean="OK Button") -> (0, 1=w198:i16)
    n113 = for {
      N: w198 -> [_]
      tunnel: w199 -> [w229]
      w233 = " " ("string")
      n114 = property on="Add comment" class="Str"("Val(Sgnl)"="" ("Value (Signaling)")) -> ()  [unwired: 2 in, 2 out]
      n115 = Get Date/Time String(want seconds? (F)=TRUE) -> (date string=w236:string, time string=w234:string)  [unwired: 2 in]
      n116 = Concatenate Strings(w236, w233, w234, w233, "Add comment") -> (w232:string)
      n117 = feedback #2() -> (w231:string[])  [unwired: 1 in]
      n118 = Build Array (concatenate)(w231, w232) -> (w230:string[])
      n119 = feedback-in #2(w230) -> ()
      n120 = Write to Text File(file (use dialog)=w229, text=w230) -> ()  [unwired: 2 in, 3 out]
    }
    n121 = call "Write To Measurement File"("Signals"=w204, "Enable"="OK Button 2", "Filename"=w12) -> ()  [unwired: 14 in, 3 out]
    "Boolean" <- "OK Button 2"
  }
